vi "screw mount detect.vi"() -> ()   [LabVIEW 2021]
doc: "This example shows how to use the Edge Tool in NI Vision. The Edge Tool finds edges (or sharp transitions in the pixels values) along a given line or ROI profile. The Edge Tool is a precursor function to many of the gauging and inspection tasks. For example, the location of the edges found along a line profile across an object can interpreted as the boundaries of the object whose dimensions have to be measured for a gauging application or the presence of a crack in the surface of an object for an inspection application."
uses:
  <vilib>/vision/Measure.llb/Edge Options.ctl
  <vilib>/vision/Measure.llb/Edge Polarity.ctl
  <vilib>/vision/Measure.llb/Straight Edge Options.ctl
  <vilib>/vision/Measure.llb/Straight Edge Process.ctl
  e759759d-0779-4853-b62f-5316b8be79e2.vi
  <vilib>/vision/NI_Vision_Development_Module.lvlib
panel:
  in  "Line Fit Options":T1={"Number of Lines"=1, "Type"=enum."Best Edge Rake", "Min. Score"=300.0, "Max. Score"=1000.0, "Orientation"=0.0, "Angle Range"=30.0, "Angle Tolerance"=1.0, "Step Size"=3, "Min. SNR (db)"=0.0, "Min. Points (%)"=25.0, "Hough Iterations"=5} {"Min. Points (%)" min=0.0 max=100.0; "Min. SNR (db)" min=0.0; "Max. Score" min=0.0 max=1024.0; "Min. Score" min=0.0 max=1024.0 step=1.0}
  out "Angle":sgl
  in  "milliseconds to wait":u32=2000
  out "PASS":bool
  out "Num":i32
  in  "Process":T3(ring)=enum."Get All Edges"
  in  "Edge Options":T4={"Edge Polarity"=0, "Kernel Size"=3, "Width"=3, "Minimum Edge Strength"=50.0, "Interpolation Type"=enum."Bilinear", "Data Processing Method"=enum."Average"} {"Edge Polarity" items=["All Edges", "Rising Edges", "Falling Edges"]; "Minimum Edge Strength" format="%.2f"; "Width" step=2; "Kernel Size" step=2}
  out "Image":T6(plugin-control)
  out "Line Profile":cluster{"x0":sgl, "dx":sgl, "Pixels Line":sgl[]}(graph)
  in  "Stop":bool
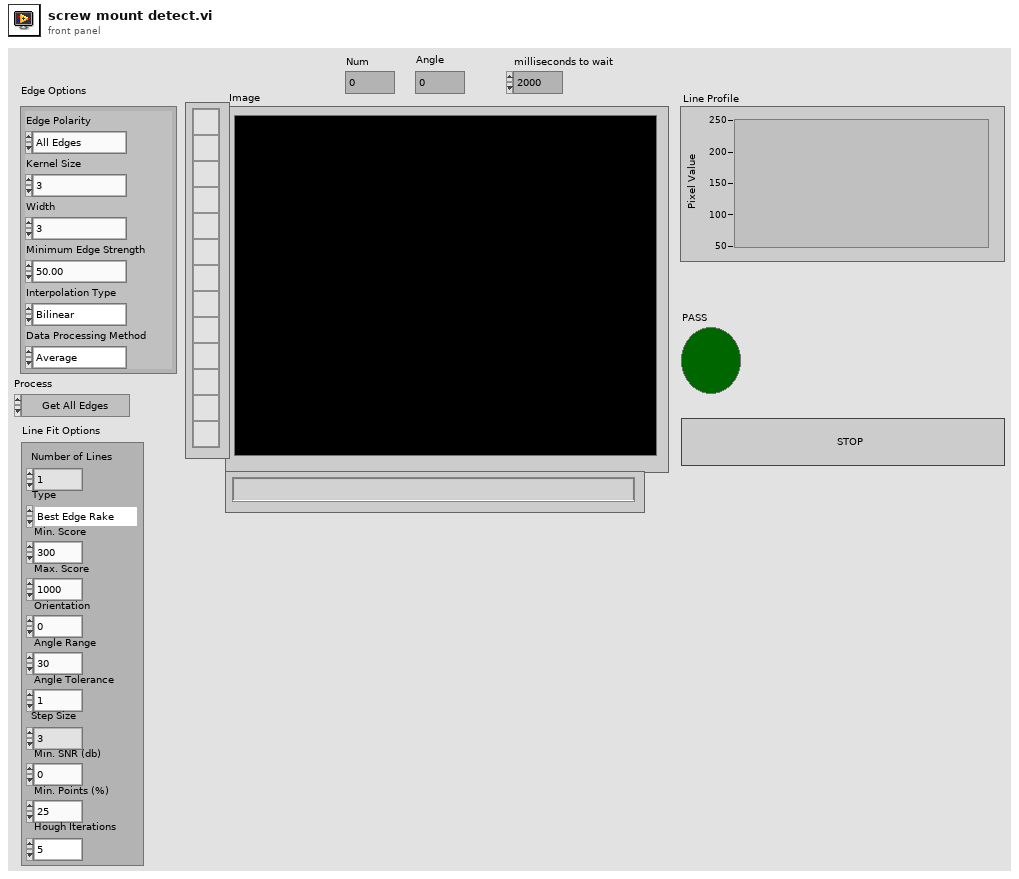
[diagram p1: front panel]
types:
  T1 = typedef "Straight Edge Options.ctl" = cluster{"Number of Lines":i32, "Type":T2, "Min. Score":dbl, "Max. Score":dbl, "Orientation":dbl, "Angle Range":dbl, "Angle Tolerance":dbl, "Step Size":u32, "Min. SNR (db)":dbl, "Min. Points (%)":dbl, "Hough Iterations":i32}
  T2 = typedef "Straight Edge Process.ctl" = enum32{"First Edge Rake", "Best Edge Rake", "Hough Edge Rake", "First Edge Projection", "Best Edge Projection"}
  T3 = enum16{"Get First Edge", "Get First + Last Edge", "Get All Edges", "Get Best Edge"}
  T4 = typedef "Edge Options.ctl" = cluster{"Edge Polarity":T5, "Kernel Size":u32, "Width":u32, "Minimum Edge Strength":sgl, "Interpolation Type":enum32{"Zero Order", "Bilinear", "Quadratic", "Cubic", "Bilinear Fixed"}, "Data Processing Method":enum32{"Average", "Median"}}
  T5 = typedef "Edge Polarity.ctl" = u32
  T6 = typedef "IMAQ Image.ctl" = refnum<image>
  T7 = typedef "IMAQ Rectangle" = cluster{"Left":i32, "Top":i32, "Right":i32, "Bottom":i32, "Rotation":dbl}
  T8 = typedef "Image Type" = u32
  T9 = typedef "ROI Descriptor" = cluster{"Global Rectangle":i32[], "Contours":cluster{"ID":enum32{"External", "Internal"}, "Type":u32, "Coordinates":i32[]}[]}
  T10 = cluster{"Search Direction":u32, "Edge Options":T4, "Show Search Area":bool, "Show Search Lines":bool, "Show Edges Found":bool, "Show Result":bool, "Search Area Color":u32, "Search Lines Color":u32, "Edge Locations Color":u32, "Result Color":u32, "Overlay Group Name":string}
  T11 = typedef "Edge New.ctl" = cluster{"Location (Pixel)":cluster{"X":sgl, "Y":sgl}, "Location (Real-World)":cluster{"X":sgl, "Y":sgl}, "Distance (Pixel)":dbl, "Distance (Real-World)":dbl, "Strength":dbl, "Noise":dbl, "Rising?":bool}
  T12 = cluster{"Point1 (Pixels)":cluster{"X":sgl, "Y":sgl}, "Point2 (Pixels)":cluster{"X":sgl, "Y":sgl}, "Point1 (Real-World)":cluster{"X":sgl, "Y":sgl}, "Point2 (Real-World)":cluster{"X":sgl, "Y":sgl}, "Angle (Pixel)":dbl, "Angle (Real-World)":dbl, "Score":dbl, "Straightness":dbl, "Average SNR (db)":dbl, "Calibration Valid":bool}[]
  T13 = cluster{"Point1 (Pixels)":cluster{"X":sgl, "Y":sgl}, "Point2 (Pixels)":cluster{"X":sgl, "Y":sgl}, "Point1 (Real-World)":cluster{"X":sgl, "Y":sgl}, "Point2 (Real-World)":cluster{"X":sgl, "Y":sgl}, "Angle (Pixel)":dbl, "Angle (Real-World)":dbl, "Score":dbl, "Straightness":dbl, "Average SNR (db)":dbl, "Calibration Valid":bool}
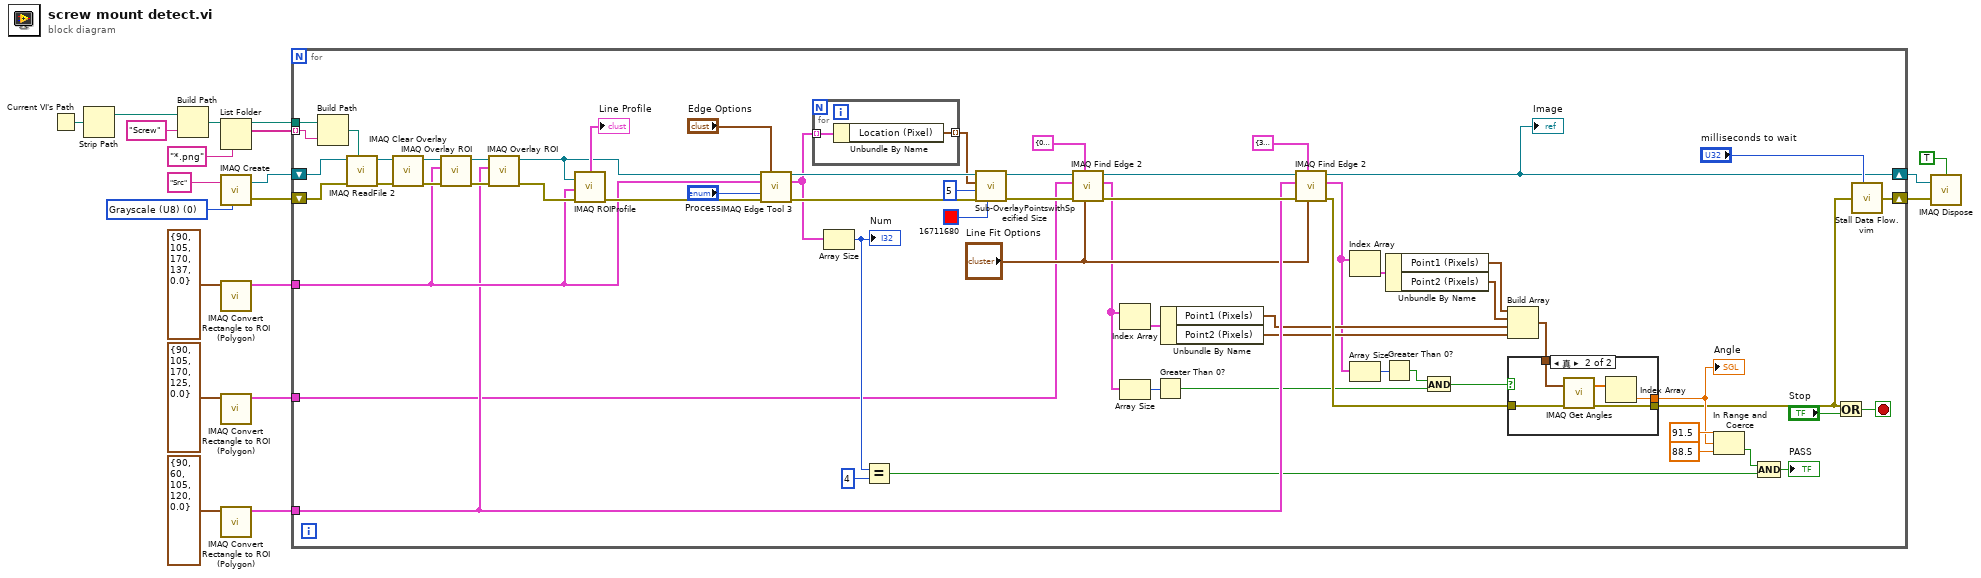
[diagram p0: block diagram]
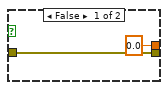
[diagram p2: hidden frame]
diagram:
  w17 = T8 0 items=["Grayscale (U8)", "Grayscale (I16)", "Grayscale (SGL)", "Complex (CSG)", "RGB (U32)", "HSL (U32)", "RGB (U64)", "Grayscale (U16)"] ("Image Type")
  n1 = Current VI's Path() -> (path=w5:path)
  n2 = Strip Path(path=w5) -> (stripped path=w4:path)  [unwired: 1 out]
  n3 = Build Path(base path=w4, name or relative path="Screw") -> (appended path=w2:path)
  n4 = List Folder(path=w2, pattern="*.png" ("类型")) -> (path out=w15:path, filenames=w16:string[])  [unwired: 2 in, 2 out]
  n5 = call "IMAQ Create"("Image Name"="Src", "Image Type"=w17) -> ("New Image"=w19:T6, "error out"=w18:errorcluster)  [unwired: 3 in]
  n6 = call "IMAQ Convert Rectangle to ROI (Polygon)"("Rectangle"=T7 {"Left"=90, "Top"=105, "Right"=170, "Bottom"=137, "Rotation"=0.0}) -> ("ROI Descriptor"=w14:T9)  [unwired: 7 in, 2 out]
  n7 = call "IMAQ Convert Rectangle to ROI (Polygon)"("Rectangle"=T7 {"Left"=90, "Top"=105, "Right"=170, "Bottom"=125, "Rotation"=0.0}) -> ("ROI Descriptor"=w6:T9)  [unwired: 7 in, 2 out]
  n8 = call "IMAQ Convert Rectangle to ROI (Polygon)"("Rectangle"=T7 {"Left"=90, "Top"=60, "Right"=105, "Bottom"=120, "Rotation"=0.0}) -> ("ROI Descriptor"=w8:T9)  [unwired: 7 in, 2 out]
  n9 = for {
    shift-right: [w51] -> w11
    shift-left: w19 -> [w82]
    shift-right: [w64] -> w12
    shift-left: w18 -> [w81]
    tunnel: w16 -> [w68] mode=indexing
    tunnel: w15 -> [w69]
    tunnel: w14 -> [w49]
    tunnel: w8 -> [w47]
    tunnel: w6 -> [w22]
    stop <- w70 stop-if-true
    n10 = Build Path(base path=w69, name or relative path=w68) -> (appended path=w67:path)
    n11 = call "IMAQ ReadFile 2"("File Path"=w67, "error in (no error)"=w81, "Image"=w82) -> ("error out"=w79:errorcluster, "Image Out"=w80:T6)  [unwired: 4 in, 3 out]
    n12 = call "IMAQ Clear Overlay"("error in (no error)"=w79, "Image"=w80) -> ("error out"=w60:errorcluster, "Image Out"=w61:T6)  [unwired: 8 in]
    n13 = call "IMAQ Overlay ROI"("error in (no error)"=w60, "ROI Descriptor"=w49, "Image"=w61) -> ("error out"=w58:errorcluster, "Image Out"=w56:T6)  [unwired: 7 in]
    n14 = call "IMAQ Overlay ROI"("error in (no error)"=w58, "ROI Descriptor"=w47, "Image"=w56) -> ("error out"=w59:errorcluster, "Image Out"=w57:T6)  [unwired: 7 in]
    n15 = call "IMAQ ROIProfile"("error in (no error)"=w59, "ROI Descriptor"=w49, "Image"=w57) -> ("error out"=w77:errorcluster, "ROI Graph"=→"Line Profile":cluster{"x0":sgl, "dx":sgl, "Pixels Line":sgl[]})  [unwired: 1 in, 3 out]
    n16 = call "IMAQ Edge Tool 3"("Image"=w57, "Edge Options"="Edge Options", "ROI Descriptor"=w49, "Process"="Process", "error in (no error)"=w77) -> ("Image (duplicate)"=w75:T6, "Edge Information"=w74:T11[], "error out"=w76:errorcluster)  [unwired: 6 in, 2 out]
    n17 = for {
      tunnel: w74 -> [w91] mode=indexing
      tunnel: [w90] -> w71 mode=indexing
      n18 = Unbundle By Name(w91) -> ("Location (Pixel)"=w90:cluster{"X":sgl, "Y":sgl})
    }
    n19 = Array Size(array=w74) -> (size(s)=w34:i32)
    "Num" <- w34
    n20 = Equal?(x=w34, y=4) -> (x = y?=w32:bool)
    n21 = call "Sub-OverlayPointswithSpecified Size.vi"("Color"=u32 16711680, "error in"=w76, "Point Diameter (5)"=u32 5, "Points"=w71, "Image In"=w75) -> ("error out"=w55:errorcluster, "Image Out"=w54:T6)  [unwired: 5 in]
    n22 = call "IMAQ Find Edge 2"("Line Fit Options"="Line Fit Options", "Options"=T10 {"Search Direction"=0, "Edge Options"={"Edge Polarity"=2, "Kernel Size"=3, "Width"=3, "Minimum Edge Strength"=50.0, "Interpolation Type"=enum."Bilinear", "Data Processing Method"=enum."Average"}, "Show Search Area"=FALSE, "Show Search Lines"=FALSE, "Show Edges Found"=FALSE, "Show Result"=TRUE, "Search Area Color"=65280, "Search Lines Color"=255, "Edge Locations Color"=16776960, "Result Color"=16711680, "Overlay Group Name"=""}, "error in (no error)"=w55, "ROI Descriptor"=w22, "Image"=w54) -> ("error out"=w53:errorcluster, "Straight Edges"=w29:T12, "Image Out"=w52:T6)  [unwired: 3 in, 1 out]
    n23 = Index Array(array=w29) -> (element=w44:T13)  [unwired: 1 in]
    n24 = Array Size(array=w29) -> (size(s)=w28:i32)
    n25 = Greater Than 0?(x=w28) -> (x > 0?=w24:bool)
    n26 = Unbundle By Name(w44) -> ("Point1 (Pixels)"=w40:cluster{"X":sgl, "Y":sgl}, "Point2 (Pixels)"=w41:cluster{"X":sgl, "Y":sgl})
    n27 = call "IMAQ Find Edge 2"("Line Fit Options"="Line Fit Options", "Options"=T10 {"Search Direction"=3, "Edge Options"={"Edge Polarity"=2, "Kernel Size"=3, "Width"=3, "Minimum Edge Strength"=50.0, "Interpolation Type"=enum."Bilinear", "Data Processing Method"=enum."Average"}, "Show Search Area"=FALSE, "Show Search Lines"=FALSE, "Show Edges Found"=FALSE, "Show Result"=TRUE, "Search Area Color"=65280, "Search Lines Color"=255, "Edge Locations Color"=16776960, "Result Color"=16711680, "Overlay Group Name"=""}, "error in (no error)"=w53, "ROI Descriptor"=w47, "Image"=w52) -> ("error out"=w45:errorcluster, "Straight Edges"=w26:T12, "Image Out"=w51:T6)  [unwired: 3 in, 1 out]
    "Image" <- w51
    n28 = Index Array(array=w26) -> (element=w43:T13)  [unwired: 1 in]
    n29 = Array Size(array=w26) -> (size(s)=w27:i32)
    n30 = Greater Than 0?(x=w27) -> (x > 0?=w25:bool)
    n31 = Unbundle By Name(w43) -> ("Point1 (Pixels)"=w38:cluster{"X":sgl, "Y":sgl}, "Point2 (Pixels)"=w39:cluster{"X":sgl, "Y":sgl})
    n32 = And(x=w25, y=w24) -> (x .and. y?=w23:bool)
    n33 = Build Array(w38, w39, w40, w41) -> (w42:cluster{"X":sgl, "Y":sgl}[])
    n34 = case shown="真" w23 {
      tunnel: w45 -> [w84 w89]
      tunnel: [w84 w88] -> w21
      tunnel: w42 -> [_ w87]
      tunnel: [sgl 0.0 ("Angle (deg)") w85] -> w30
      frame False {
      }
      frame True {
        n35 = call "IMAQ Get Angles"("error in (no error)"=w89, "Points"=w87) -> ("error out"=w88:errorcluster, "Angles (deg)"=w86:sgl[])  [unwired: 3 in, 1 out]
        n36 = Index Array(array=w86) -> (element=w85:sgl)  [unwired: 1 in]
      }
    }
    "Angle" <- w30
    n37 = In Range and Coerce(upper limit=sgl 91.5 ("上限"), x=w30, lower limit=sgl 88.5 ("下限")) -> (In Range?=w35:bool)  [unwired: 1 out]
    n38 = Compound Arithmetic op=AND ("复合运算")(w35, w32) -> (→"PASS":bool)
    n39 = Or(x=w21, y="Stop") -> (x .or. y?=w70:bool)
    n40 = call "Stall Data Flow.vim"("value in"=w21, "milliseconds to wait"="milliseconds to wait") -> ("value out"=w64:errorcluster)  [unwired: 1 out]
  }
  n41 = call "IMAQ Dispose"("All Images? (No)"=TRUE, "Image"=w11, "error in (no error)"=w12) -> ()  [unwired: 3 in, 1 out]
